vi "Set Parent Visible.vi"(8 "error in (no error)":errorcluster, 10 "Parent visible? [T]":bool=TRUE, 11 "IContainer in":refnum<class "IContainer.lvclass">) -> (0 "error out":errorcluster, 3 "IContainer out":refnum<class "IContainer.lvclass">)   [LabVIEW 2021, in "IContainer.lvclass"]
doc: "Copyright 2018, Wiebe Walstra, wiebe@carya.nl."
uses:
  IContainer.lvclass
  IContainer.lvclass/IContainer.ctl
  IObject.lvclass
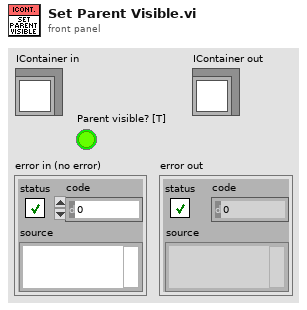
[diagram p1: front panel]
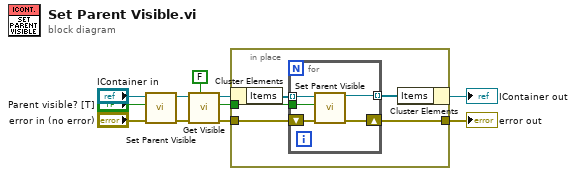
[diagram p0: block diagram]
diagram:
  n1 = call-parent "Set Parent Visible.vi"("error in (no error)"="error in (no error)", "Parent visible? [T]"="Parent visible? [T]", "IObject in"="IContainer in") -> ("error out"=w5:errorcluster, "IObject out"=w3:refnum<class "IContainer.lvclass">)  [unwired: 7 in]
  n2 = call-dynamic "Get Visible.vi"("Hide if children are hidden? [T]"=FALSE, "error in (no error)"=w5, "IContainer in"=w3) -> ("error out"=w6:errorcluster, "Visible?"=w8:bool, "IContainer out"=w7:refnum<class "IContainer.lvclass">)  [unwired: 5 in, 1 out]
  n3 = in-place {
    in-place-border: [w16] -> w4
    in-place-border: w6 -> [w15]
    in-place-border: w8 -> [w13]
    n4 = in-place-cluster #1(w7) -> ("Items"=w14:refnum<class "IObject.lvclass">[])
    n5 = for {
      tunnel: [w17] -> w12 mode=indexing
      tunnel: w14 -> [w20] mode=indexing
      shift-right: [w18] -> w16
      shift-left: w15 -> [w21]
      tunnel: w13 -> [w19]
      n6 = call-dynamic "Set Parent Visible.vi"("error in (no error)"=w21, "Parent visible? [T]"=w19, "IObject in"=w20) -> ("error out"=w18:errorcluster, "IObject out"=w17:refnum<class "IObject.lvclass">)  [unwired: 7 in]
    }
    n7 = in-place-cluster #1("Items"=w12) -> (→"IContainer out":refnum<class "IContainer.lvclass">)
  }
  "error out" <- w4
